vi "Save Image to raw.vi"(8 "error in":errorcluster, 10 "file path":path, 11 "Last displayed image data in":u32[](array[numeric])) -> (0 "error out":errorcluster)   [LabVIEW 2025, in "Automotive Vision.lvclass"]
doc: "Saves the current frame to a raw file."
uses:
  Automotive Vision.lvclass
  Automotive Vision.lvclass/Automotive Vision.ctl
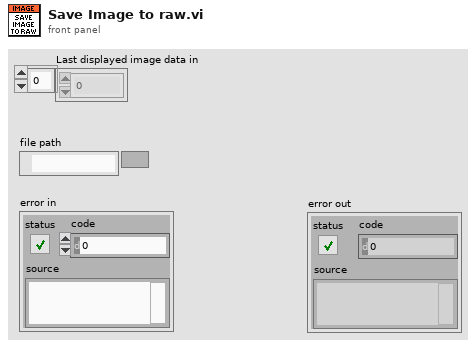
[diagram p1: front panel]
types:
  T1 = enum16{"open", "replace", "create", "open or create", "replace or create", "replace or create with confirmation"}
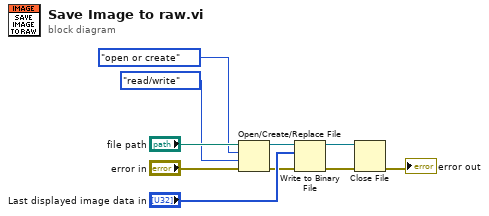
[diagram p0: block diagram]
diagram:
  n1 = Open/Create/Replace File(file path (use dialog)="file path", error in="error in", operation (0:open)=T1."open or create", access (0:read/write)=enum16{"read/write", "read-only", "write-only"}."read/write") -> (refnum out=w7:refnum<file>, error out=w3:errorcluster)  [unwired: 2 in, 1 out]
  n2 = Write to Binary File(file (use dialog)=w7, data="Last displayed image data in", error in=w3) -> (refnum out=w5:refnum<file>, error out=w2:errorcluster)  [unwired: 3 in, 1 out]
  n3 = Close File(refnum=w5, error in=w2) -> (error out=→"error out":errorcluster)  [unwired: 1 out]
